vi "Google Spreadsheet Uploader LaunchPad-v4.vi"(7 "Status?":string="Enable", 9 "Inputs String Array":string[](array[string]), 11 "formkey":string="dFNhUnAta3JpbUNkdlNvUmFVeTFBdVE6MQ") -> (1 "fail? read":bool, 3 "fail? write":bool)   [LabVIEW 2011]
panel:
  out "array index":string[](array[string])
  out "data":string
  # "note for VPN uploader\nformkey=dENGX2UtWTk4MVg2VElzUENMVHpSN1E6MQ\nhttps://docs.google.com/spreadsheet/ccc?key=0ApN06iNJ4ajEdENGX2UtWTk4MVg2VElzUENMVHpSN1E&hl=en_US#gid=0"
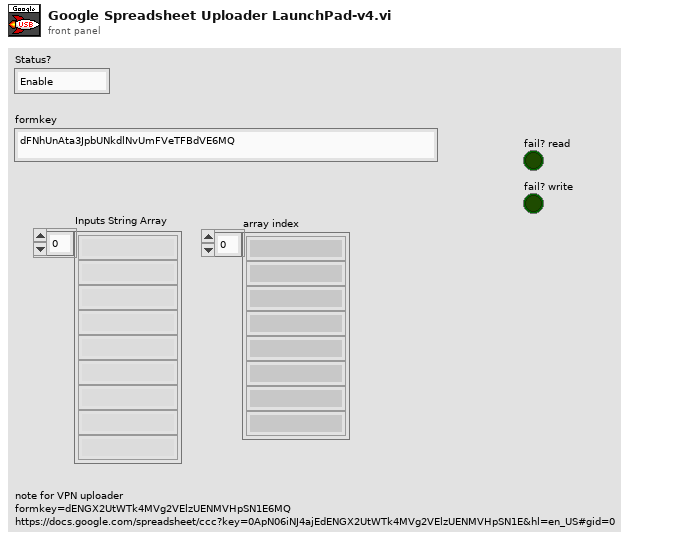
[diagram p1: front panel]
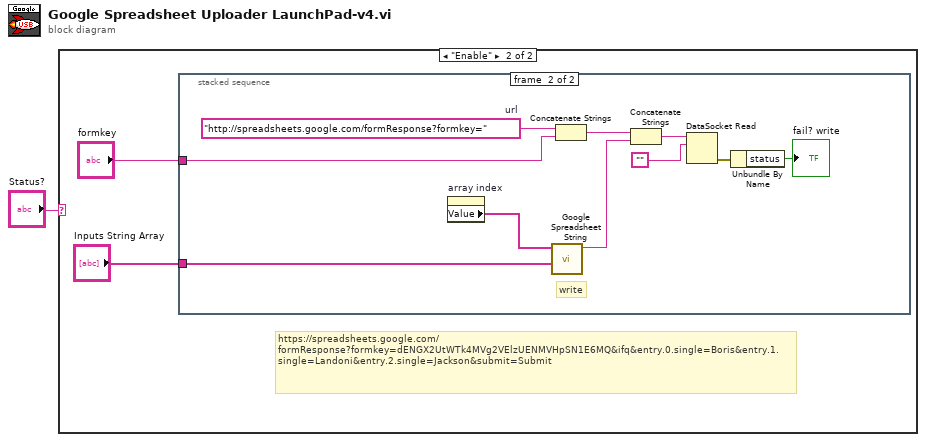
[diagram p0: block diagram]
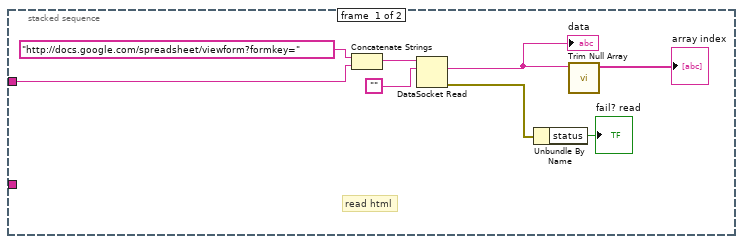
[diagram p3: hidden frame]
diagram:
  n1 = case shown="\"Enable\"" "Status?" {
    frame "Disable", Default {
    }
    frame "Enable" {
      # "https://spreadsheets.google.com/formResponse?formkey=dENGX2UtWTk4MVg2VElzUENMVHpSN1E6MQ&ifq&entry.0.single=Boris&entry.1.single=Landoni&entry.2.single=Jackson&submit=Submit"
      n2 = stacked-sequence {
        tunnel: "formkey" -> [w10 w19]
        tunnel: "Inputs String Array" -> [_ w13]
        frame #0 {
          # "read html"
          n3 = Concatenate Strings("http://docs.google.com/spreadsheet/viewform?formkey=", w10) -> (w9:string)
          n4 = DataSocket Read(10:"", 11:w9) -> (0:w6:errorcluster, 2:w5:string)  [unwired: 1 in, 7 out]
          "data" <- w5
          n5 = Unbundle By Name(w6) -> ("status"=→"fail? read":bool)
          n6 = call "Trim Null Array.vi"("String"=w5) -> ("output array"=→"array index":string[])  [unwired: 10 in]
        }
        frame #1 {
          w20 = "http://spreadsheets.google.com/formResponse?formkey="  # url
          # "write"
          n7 = property on="array index" class="Arr (strict)"() -> ("Value"=w12:string[])  [unwired: 2 in, 2 out]
          n8 = call "Google Spreadsheet String.vi"("Array Value"=w13, "Array Index"=w12) -> ("Output string"=w14:string)  [unwired: 7 in, 2 out]
          n9 = Concatenate Strings(w20, w19) -> (w18:string)
          n10 = Concatenate Strings(w18, w14) -> (w16:string)
          n11 = DataSocket Read(10:"", 11:w16) -> (0:w17:errorcluster)  [unwired: 1 in, 8 out]
          n12 = Unbundle By Name(w17) -> ("status"=→"fail? write":bool)
        }
      }
    }
  }
